vi "Create.vi"(8 "error in (no error)":errorcluster) -> (0 "error out":errorcluster, 3 "Log file path":path)   [LabVIEW 2018, in "app_log.lvlib"]
doc: "Creates the \"Knight Tour Log\" file. The knight tours found by the program are stored in this file."
uses:
  app_log.lvlib
  text_file/text_file.lvlib
panel:
  # "Development\ncontrols/indicators useful for development and testing, but which are not outputs of the VI"
  # "Input\nInputs to the VI"
  # "Output\nOutputs of the VI"
  # "Description\n\nBlank VI with error handling case. \n\nSummarize the use of this VI in this space."
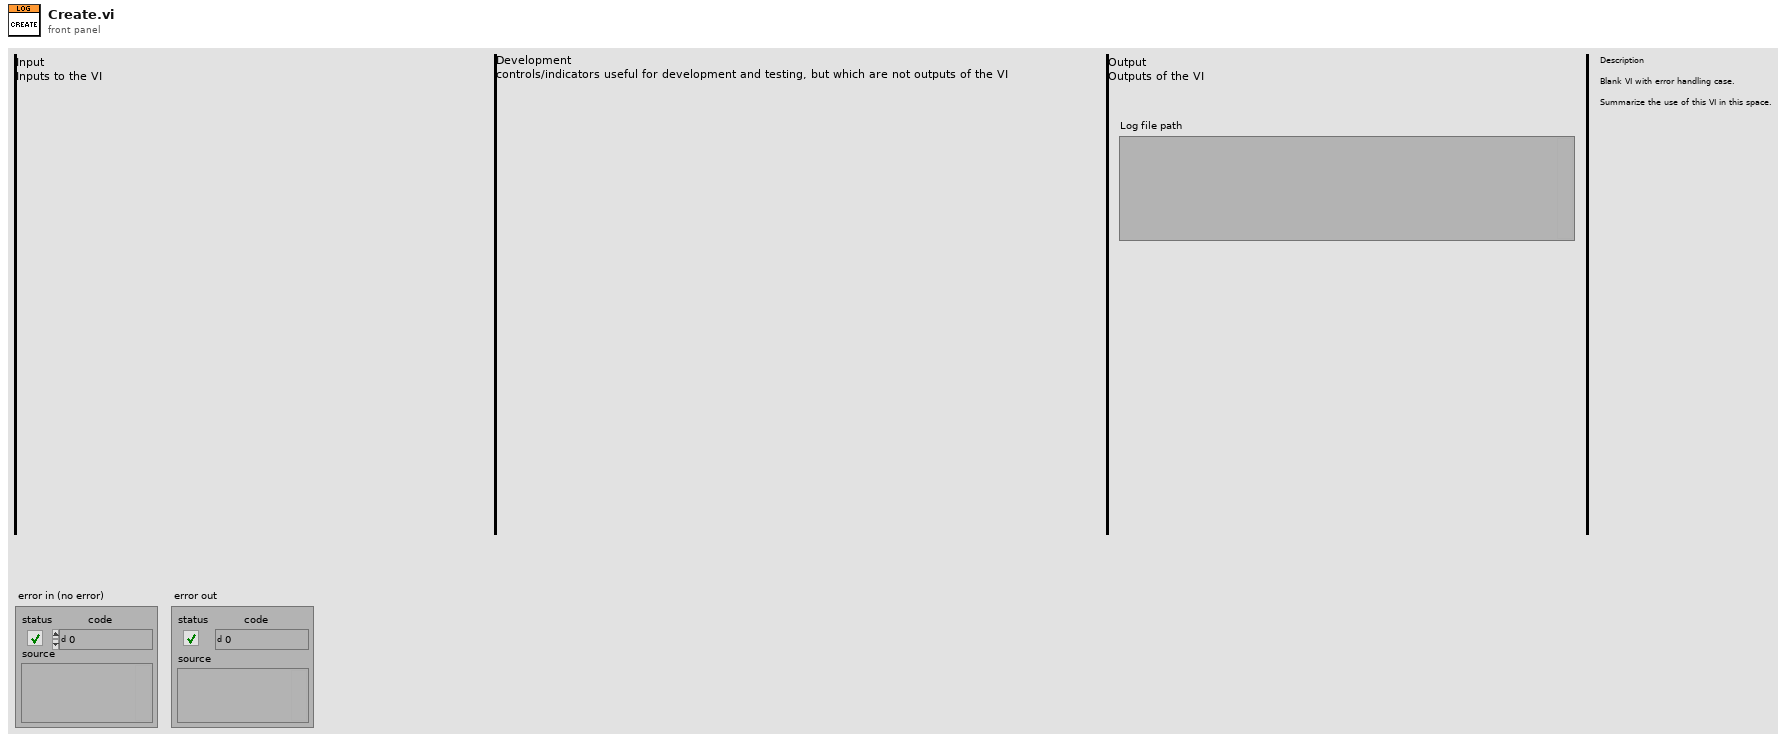
[diagram p1: front panel]
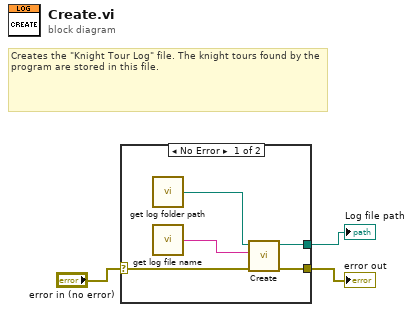
[diagram p0: block diagram]
diagram:
  # "Creates the \"Knight Tour Log\" file. The knight tours found by the program are stored in this file."
  n1 = case shown="No Error" "error in (no error)" {
    selector: "error in (no error)" -> [w8 w9]
    tunnel: [w7 w9] -> w2
    tunnel: [w4 _] -> w1
    frame No Error {
      n2 = call "get log folder path.vi"() -> ("log folder path"=w6:path)
      n3 = call "get log file name.vi"() -> ("log file name (excluding extension)"=w5:string)
      n4 = call "Create.vi"("error in (no error)"=w8, "File name (exclude extension)"=w5, "Folder (create file inside this folder)"=w6) -> ("error out"=w7:errorcluster, "Log file path"=w4:path)  [unwired: 7 in]
    }
    frame Error {
    }
  }
  "error out" <- w2
  "Log file path" <- w1
